vi "断电保存全局.vi"() -> ()   [LabVIEW 2016, in "Alarm interface.lvlib"]
uses:
  Alarm interface.lvlib
panel:
  out "三级报警":string[][](array[string])
  out "二级报警":string[][](array[string])
  out "一级报警":string[][](array[string])
  in  "短信语音用户列表":string[][](array[string])
  in  "报警定义表":string[][](array[string])=[["一级", "短信 电话 微信", "0-1000"], ["二级", "短信 电话 微信", "1001-2000"], ["三级", "短信 电话 微信", "2001-3000"]]
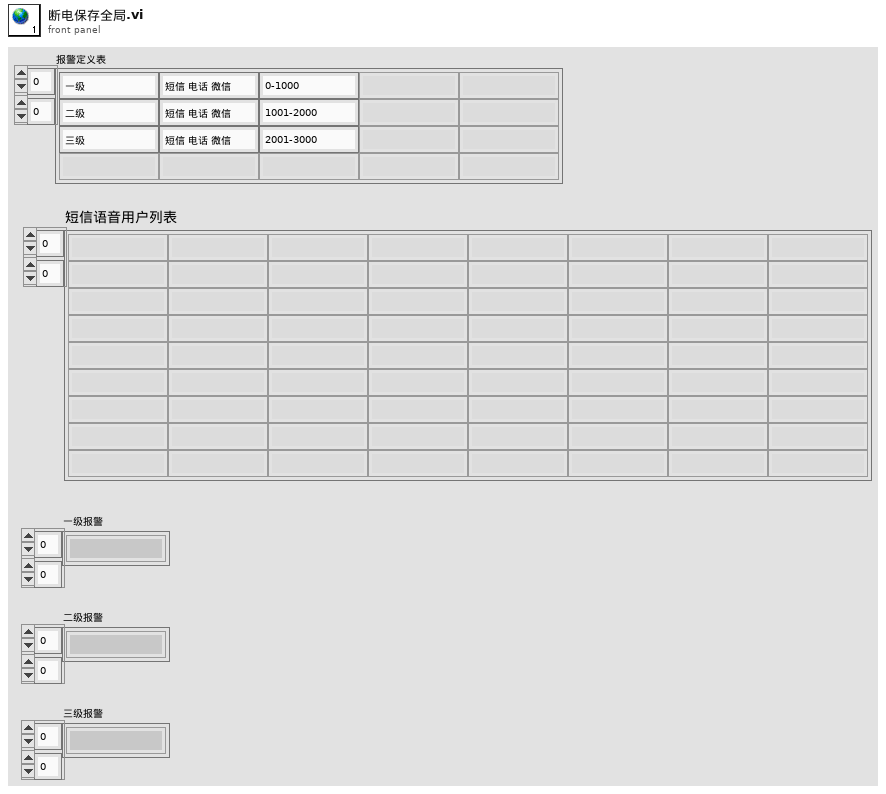
[diagram p1: front panel]
diagram:
